vi "五参数水样测试.vi"(11 "启动参数":T1={"测量模式"="", "数据类型"="N"}) -> ()   [LabVIEW 2016, in "斯坦道原位多参数.lvlib"]
panel:
  out "Elapsed Time (s)":dbl caption="已用时间(s)"
  out "状态":string
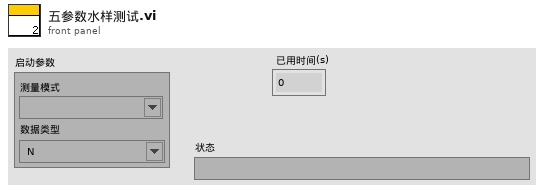
[diagram p1: front panel]
types:
  T1 = typedef "斯坦道原位多参数.lvlib/水样测试启动自定义输入参数.ctl" = cluster{"测量模式":string, "数据类型":string}
  T2 = cluster{"时间标识":timestamp, "设备":string, "日志信息":string, "流程参数":string}
  T3 = cluster{"水温":bool, "pH":bool, "DO":bool, "DOper":bool, "电导率":bool, "ORP":bool, "浊度":bool, "叶绿素a":bool, "藻密度":bool}
  T4 = typedef "原位多参数全参数字段定义.ctl" = cluster{"时间":timestamp, "水温":dbl, "pH":dbl, "DO":dbl, "DO%":dbl, "电导率":dbl, "ORP":dbl, "浊度":dbl, "叶绿素a":dbl, "藻密度":dbl}
  T5 = cluster{"系统时间":timestamp, "工作状态":u16, "测量模式":u16, "告警代码":enum16{"无告警", "缺试剂告警", "缺水样告警", "缺蒸馏水告警", "缺标液告警", "仪表漏液告警", "标定异常告警", "超量程告警", "加热异常", "低试剂预警", "超上限告警", "超下限告警", "仪表内部其他异常", "滴定异常告警", "电极异常告警", "量程切换告警", "参数设置告警", "PH电极电位异常", "电导率电极异常", "浊度光度异常", "溶解氧电极异常", "溶解氧光强异常", "温度异常告警", "PH异常告警", "溶解氧异常告警", "电导率异常告警", "浊度异常告警", "叶绿素异常告警", "藻密度异常告警", "蓝绿藻异常告警", "ORP异常告警", "氨氮异常告警", "清洁刷异常告警", "SD卡异常告警", "蓝牙异常告警", "Wifi异常告警", "流程异常告警"}, "故障代码":enum16{"无故障", "电机故障", "温度故障", "通讯故障", "滴定故障"}, "日志代码":u16, "软件版本":string}
  T6 = cluster{"水温":dbl, "pH":dbl, "DO":dbl, "Cond":dbl, "Turb":dbl, "叶绿素":dbl, "藻密度":dbl, "蓝绿藻":dbl, "ORP":dbl, "NH3N":dbl}
  T7 = cluster{"因子编码":string, "单位":string, "标样参考值":sgl, "水样数据时间":timestamp, "水样实测值":sgl, "水样数据标识":string, "K":sgl, "B":sgl, "T":sgl, "H":sgl, "水深":sgl, "探头温度":sgl, "信号值":sgl}
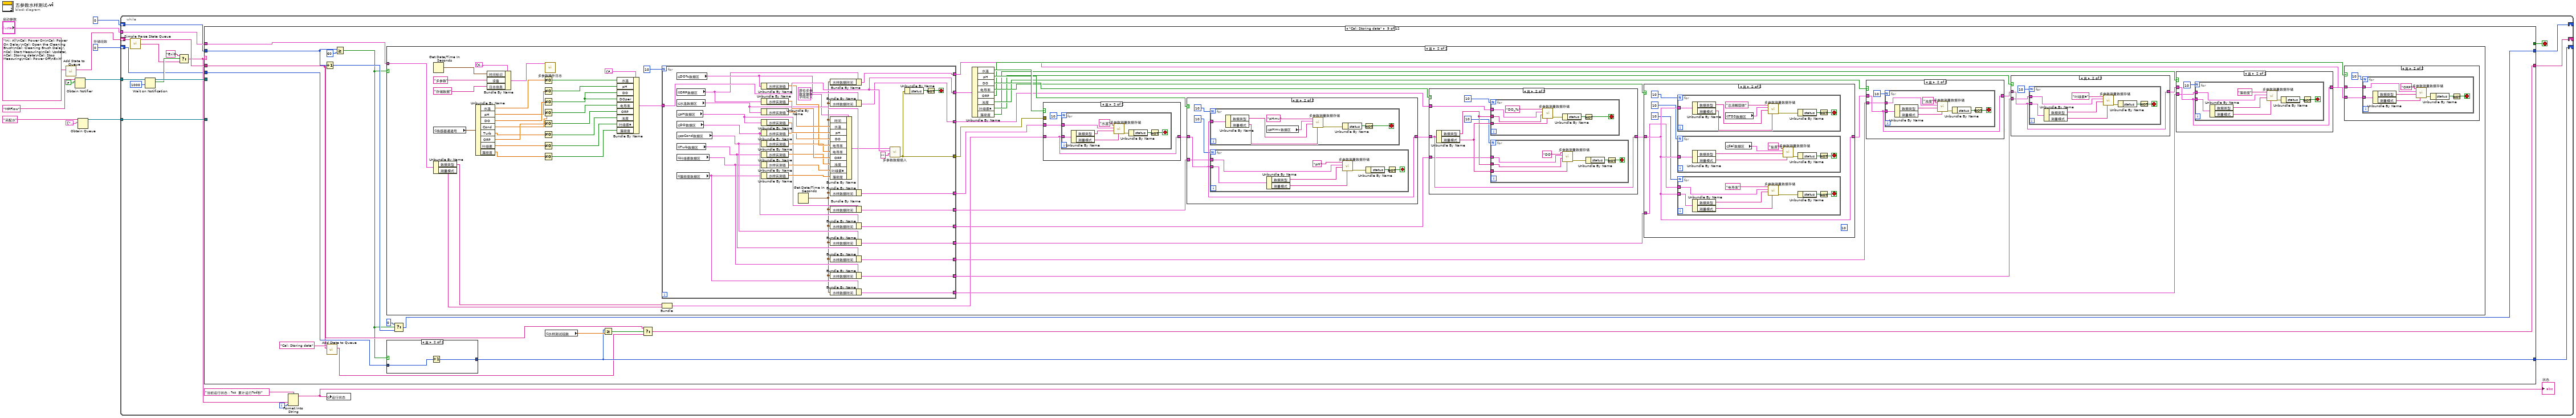
[diagram p0: block diagram]
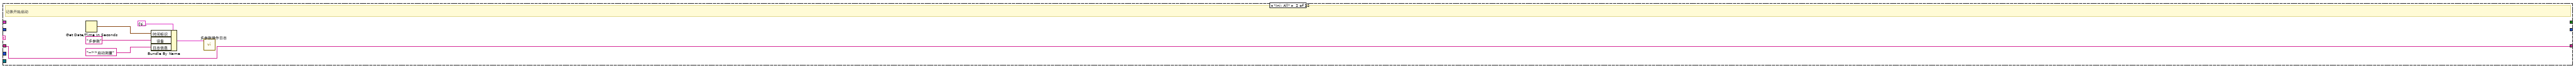
[diagram p3: hidden frame]
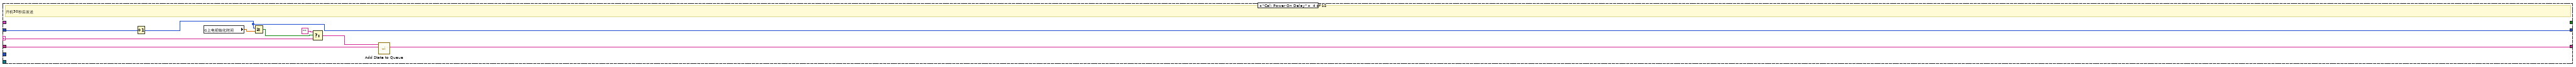
[diagram p5: hidden frame]
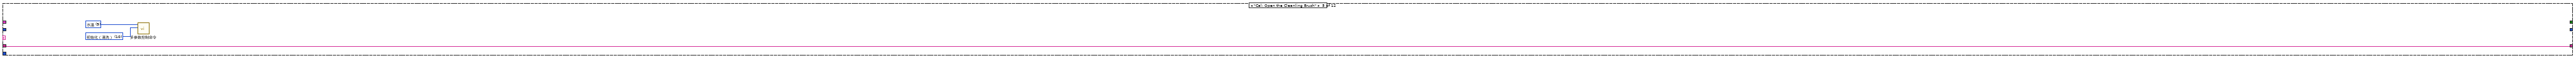
[diagram p6: hidden frame]
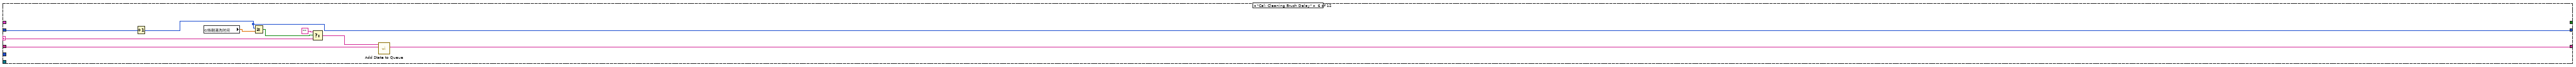
[diagram p7: hidden frame]
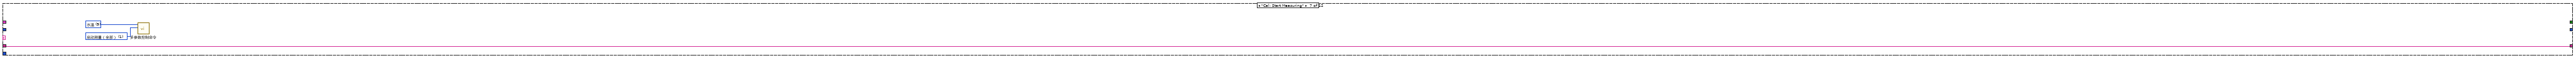
[diagram p8: hidden frame]
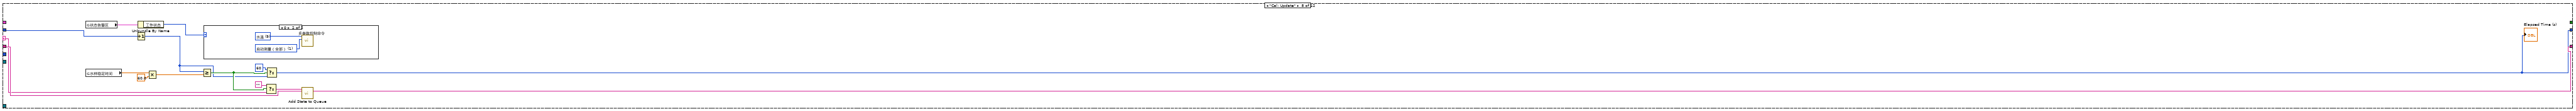
[diagram p9: hidden frame]
diagram:
  w1 = 0  # 存储组数
  n1 = call "Add State to Queue.vi"("State(s) In (\"\")"="Ini: All\nCal: Power On\nCal: Power On Delay\nCal: Open the Cleaning Brush\nCal: Cleaning Brush Delay\nCal: Start Measuring\nCal: Update\nCal: Storing data\nCal: Stop Measuring\nCal: Power Off\nExit" ("State(s) In (\"\")")) -> ("States Out"=w10:string)  [unwired: 14 in]
  n2 = Obtain Notifier(name (unnamed)="MPFlow" ("名称（未命名）"), notification data type=FALSE) -> (notifier out=w4:refnum<notifier>)  [unwired: 2 in, 2 out]
  n3 = Obtain Queue(name (unnamed)="采配水" ("名称（未命名）"), element data type=cluster{"命令":string, "数据":variant} {"命令"="", "数据"=variant}) -> (queue out=w5:refnum<queue>)  [unwired: 3 in, 2 out]
  n4 = while {
    shift-right: [w29] -> _
    shift-left: w10 -> [w31]
    tunnel: w5 -> [w28]
    tunnel: w4 -> [w27]
    tunnel: "启动参数" -> [w26]
    shift-right: [w14] -> _
    shift-left: 0 -> [w15]
    shift-right: [w13] -> _
    shift-left: w1 -> [w12]
    i -> [w24]
    stop <- w22 stop-if-true
    n5 = call "Simple Parse State Queue.vi"("State Queue"=w31) -> ("Remain States"=w30:string, "Next State"=w17:string)  [unwired: 13 in]
    n6 = Wait on Notification(notifier=w27, timeout in ms (-1)=1000 ("超时毫秒(-1)")) -> (notifier out=w21:refnum<notifier>, notification=w19:bool)  [unwired: 2 in, 2 out]
    n7 = Select(t="Exit" ("State(s) In (\"\")"), s=w19, f=w17) -> (s? t:f=w16:string)
    n8 = case shown="\"Cal: Storing data\"" w16 {
      selector: w16 -> [_ _ _ w46 _ w56 _ w74 _ _ _ _]
      tunnel: w30 -> [w32 w38 w39 w48 w51 w60 w61 w75 w87 w321 w330 w333]
      tunnel: [w32 w38 w39 w47 w51 w59 w61 w71 w89 w321 w330 w333] -> w29
      tunnel: w28 -> [_ _ _ _ _ _ _ _ _ _ _ w332]
      tunnel: w21 -> [_ _ _ _ _ _ _ _ _ _ _ w331]
      tunnel: w26 -> [_ _ _ _ _ _ _ _ w95 _ _ _]
      tunnel: [_ _ _ _ _ _ _ _ _ _ _ TRUE] -> w22
      tunnel: w15 -> [_ _ _ w43 _ w55 _ w70 w86 _ _ _]
      tunnel: [_ _ _ w42 _ w54 _ w65 w83 _ _ _] -> w14
      tunnel: w12 -> [_ _ _ _ _ _ _ _ w94 _ _ _]
      tunnel: [_ _ _ _ _ _ _ _ w91 _ _ _] -> w13
      frame Default {
      }
      frame "Ini: All" {
        # "记录开始启动"
        n9 = Get Date/Time In Seconds() -> (seconds since 1Jan1904=w34:timestamp)
        n10 = Bundle By Name(cluster=T2 {"时间标识"=timestamp(0 s since 1904-01-01), "设备"="", "日志信息"="", "流程参数"=""} ("data in"), "时间标识"=w34, "设备"="多参数", "日志信息"="-->>启动测量") -> (w35:T2)
        n11 = call "多参数操作日志.vi"("data"=w35) -> ()  [unwired: 10 in, 1 out]
      }
      frame "Cal: Power On" {
      }
      frame "Cal: Power On Delay" {
        # "开机30秒后发送"
        n12 = Increment(x=w43) -> (x+1=w42:i32)
        n13 = global read "多参数断电保存全局变量.vi" "上电初始化时间"() -> (w40:dbl)
        n14 = Greater Or Equal?(x=w42, y=w40) -> (x >= y?=w41:bool)
        n15 = Select(t="", s=w41, f=w46) -> (s? t:f=w44:string)
        n16 = call "Add State to Queue.vi"("State(s) In Front (\"\")"=w44, "State(s) In (\"\")"=w48) -> ("States Out"=w47:string)  [unwired: 13 in]
      }
      frame "Cal: Open the Cleanling Brush" {
        w50 = u16 10 items=["启动测量（全部）"=1, "初始化（清洗）"=10, "停止测量（全部）"=11, "校时"=13, "启动测量（单个传感器）"=19, "停止测量（单个传感器）"=20] ("控制命令")
        w49 = u16 9 items=["氨氮"=3, "水温"=9, "pH值"=10, "溶解氧"=11, "电导率"=12, "浊度"=13, "叶绿素a"=14, "藻密度"=15, "蓝绿藻"=16, "氧化还原电位"=17, "溶解氧%"=18, "盐度"=19] ("站号")
        n17 = call "多参数控制命令.vi"("控制命令"=w50, "站号"=w49) -> ()  [unwired: 9 in, 1 out]
      }
      frame "Cal: Cleaning Brush Delay" {
        n18 = Increment(x=w55) -> (x+1=w54:i32)
        n19 = global read "多参数断电保存全局变量.vi" "转刷清洗时间"() -> (w52:dbl)
        n20 = Greater Or Equal?(x=w54, y=w52) -> (x >= y?=w53:bool)
        n21 = Select(t="", s=w53, f=w56) -> (s? t:f=w57:string)
        n22 = call "Add State to Queue.vi"("State(s) In Front (\"\")"=w57, "State(s) In (\"\")"=w60) -> ("States Out"=w59:string)  [unwired: 13 in]
      }
      frame "Cal: Start Measuring" {
        w63 = u16 1 items=["启动测量（全部）"=1, "初始化（清洗）"=10, "停止测量（全部）"=11, "校时"=13, "启动测量（单个传感器）"=19, "停止测量（单个传感器）"=20] ("控制命令")
        w62 = u16 9 items=["氨氮"=3, "水温"=9, "pH值"=10, "溶解氧"=11, "电导率"=12, "浊度"=13, "叶绿素a"=14, "藻密度"=15, "蓝绿藻"=16, "氧化还原电位"=17, "溶解氧%"=18, "盐度"=19] ("站号")
        n23 = call "多参数控制命令.vi"("控制命令"=w63, "站号"=w62) -> ()  [unwired: 9 in, 1 out]
      }
      frame "Cal: Update" {
        n24 = global read "多参数全局变量.vi" "状态告警区"() -> (w77:T5)
        n25 = global read "多参数断电保存全局变量.vi" "水样稳定时间"() -> (w68:dbl)
        n26 = Increment(x=w70) -> (x+1=w66:i32)
        n27 = Unbundle By Name(w77) -> ("工作状态"=w78:u16)
        n28 = Multiply(x=w68, y=60.0) -> (x*y=w69:dbl)
        n29 = Greater Or Equal?(x=w66, y=w69) -> (x >= y?=w67:bool)
        n30 = case shown="0" w78 {
          frame Default {
          }
          frame 0 {
            w79 = u16 1 items=["启动测量（全部）"=1, "初始化（清洗）"=10, "停止测量（全部）"=11, "校时"=13, "启动测量（单个传感器）"=19, "停止测量（单个传感器）"=20] ("控制命令")
            w80 = u16 9 items=["氨氮"=3, "水温"=9, "pH值"=10, "溶解氧"=11, "电导率"=12, "浊度"=13, "叶绿素a"=14, "藻密度"=15, "蓝绿藻"=16, "氧化还原电位"=17, "溶解氧%"=18, "盐度"=19] ("站号")
            n31 = call "多参数控制命令.vi"("控制命令"=w79, "站号"=w80) -> ()  [unwired: 9 in, 1 out]
          }
        }
        n32 = Select(t="", s=w67, f=w74) -> (s? t:f=w73:string)
        n33 = Select(t=60, s=w67, f=w66) -> (s? t:f=w65:i32)
        "Elapsed Time (s)" <- w65
        n34 = call "Add State to Queue.vi"("State(s) In Front (\"\")"=w73, "State(s) In (\"\")"=w75) -> ("States Out"=w71:string)  [unwired: 13 in]
      }
      frame "Cal: Storing data" {
        n35 = Increment(x=w86) -> (x+1=w84:i32)
        n36 = call "Add State to Queue.vi"("State(s) In Front (\"\")"="Cal: Storing data" ("State(s) In Front (\"\")"), "State(s) In (\"\")"=w87) -> ("States Out"=w88:string)  [unwired: 13 in]
        n37 = Greater Or Equal?(x=w86, y=60) -> (x >= y?=w81:bool)
        n38 = case shown="真" w81 {
          tunnel: w95 -> [_ w139]
          frame False {
          }
          frame True {
            n39 = Get Date/Time In Seconds() -> (seconds since 1Jan1904=w148:timestamp)
            n40 = global read "多参数全局变量.vi" "传感器通道号"() -> (w121:T6)
            n41 = Unbundle By Name(w139) -> ("数据类型"=w140:string, "测量模式"=w141:string)
            n42 = Unbundle By Name(w121) -> ("水温"=w119:dbl, "pH"=w122:dbl, "DO"=w124:dbl, "Cond"=w126:dbl, "Turb"=w128:dbl, "ORP"=w130:dbl, "叶绿素"=w132:dbl, "藻密度"=w133:dbl)
            n43 = Bundle By Name(cluster=T2 {"时间标识"=timestamp(0 s since 1904-01-01), "设备"="", "日志信息"="", "流程参数"=""} ("data in"), "时间标识"=w148, "设备"="多参数", "日志信息"="存储数据") -> (w149:T2)
            n44 = Not Equal To 0?(x=w119) -> (x != 0?=w120:bool)
            n45 = Not Equal To 0?(x=w122) -> (x != 0?=w123:bool)
            n46 = Not Equal To 0?(x=w124) -> (x != 0?=w125:bool)
            n47 = Not Equal To 0?(x=w126) -> (x != 0?=w127:bool)
            n48 = Not Equal To 0?(x=w130) -> (x != 0?=w131:bool)
            n49 = Not Equal To 0?(x=w128) -> (x != 0?=w129:bool)
            n50 = Not Equal To 0?(x=w132) -> (x != 0?=w134:bool)
            n51 = Not Equal To 0?(x=w133) -> (x != 0?=w135:bool)
            n52 = call "多参数操作日志.vi"("data"=w149) -> ()  [unwired: 10 in, 1 out]
            n53 = Bundle By Name(cluster=T3 {"水温"=FALSE, "pH"=FALSE, "DO"=FALSE, "DOper"=FALSE, "电导率"=FALSE, "ORP"=FALSE, "浊度"=FALSE, "叶绿素a"=FALSE, "藻密度"=FALSE} ("columns enable"), "水温"=w120, "pH"=w123, "DO"=w125, "DOper"=w125, "电导率"=w127, "ORP"=w131, "浊度"=w129, "叶绿素a"=w134, "藻密度"=w135) -> (w117:T3)
            n54 = for {
              N: 10 -> [_]
              tunnel: [w186] -> w136
              tunnel: w117 -> [w185]
              tunnel: [w185] -> w108
              tunnel: [w161] -> w107
              tunnel: [w160] -> w106
              tunnel: [w159] -> w105
              tunnel: [w162] -> w104
              tunnel: [w158] -> w103
              tunnel: [w166] -> w102
              tunnel: [w163] -> w101
              tunnel: [w164] -> w100
              tunnel: [w165] -> w99
              stop <- w187 stop-if-true
              n55 = global read "多参数全局变量.vi" "DO%数据区"() -> (w172:T7)
              n56 = global read "多参数全局变量.vi" "ORP数据区"() -> (w170:T7)
              n57 = global read "多参数全局变量.vi" "水温数据区"() -> (w175:T7)
              n58 = global read "多参数全局变量.vi" "pH数据区"() -> (w174:T7)
              n59 = global read "多参数全局变量.vi" "DO数据区"() -> (w173:T7)
              n60 = global read "多参数全局变量.vi" "spCond数据区"() -> (w171:T7)
              n61 = global read "多参数全局变量.vi" "Turb数据区"() -> (w169:T7)
              n62 = global read "多参数全局变量.vi" "叶绿素数据区"() -> (w168:T7)
              n63 = global read "多参数全局变量.vi" "藻密度数据区"() -> (w167:T7)
              n64 = Unbundle By Name(w172) -> ("水样实测值"=w181:sgl)
              n65 = Unbundle By Name(w170) -> ("水样实测值"=w179:sgl)
              n66 = Unbundle By Name(w175) -> ("水样实测值"=w184:sgl)
              n67 = Unbundle By Name(w174) -> ("水样实测值"=w183:sgl)
              n68 = Unbundle By Name(w173) -> ("水样实测值"=w182:sgl)
              n69 = Unbundle By Name(w171) -> ("水样实测值"=w180:sgl)
              n70 = Unbundle By Name(w169) -> ("水样实测值"=w178:sgl)
              n71 = Unbundle By Name(w168) -> ("水样实测值"=w177:sgl)
              n72 = Unbundle By Name(w167) -> ("水样实测值"=w176:sgl)
              n73 = Get Date/Time In Seconds() -> (seconds since 1Jan1904=w157:timestamp)
              n74 = Bundle By Name(cluster=w170, "水样数据时间"=w157) -> (w166:T7)
              n75 = Bundle By Name(cluster=w172, "水样数据时间"=w157) -> (w162:T7)
              n76 = Bundle By Name(cluster=T4 {"时间"=timestamp(0 s since 1904-01-01), "水温"=0.0, "pH"=0.0, "DO"=0.0, "DO%"=0.0, "电导率"=0.0, "ORP"=0.0, "浊度"=0.0, "叶绿素a"=0.0, "藻密度"=0.0} ("data in"), "时间"=w157, "水温"=w184, "pH"=w183, "DO"=w182, "电导率"=w181, "电导率"=w180, "ORP"=w179, "浊度"=w178, "叶绿素a"=w177, "藻密度"=w176) -> (w155:T4)
              n77 = Bundle By Name(cluster=w175, "水样数据时间"=w157) -> (w161:T7)
              n78 = Bundle By Name(cluster=w174, "水样数据时间"=w157) -> (w160:T7)
              n79 = Bundle By Name(cluster=w173, "水样数据时间"=w157) -> (w159:T7)
              n80 = Bundle By Name(cluster=w171, "水样数据时间"=w157) -> (w158:T7)
              n81 = Bundle By Name(cluster=w169, "水样数据时间"=w157) -> (w163:T7)
              n82 = Bundle By Name(cluster=w168, "水样数据时间"=w157) -> (w164:T7)
              n83 = Bundle By Name(cluster=w167, "水样数据时间"=w157) -> (w165:T7)
              n84 = call "多参数数据插入.vi"("编号"="", "columns enable"=w185, "data in"=w155) -> ("error out"=w186:errorcluster)  [unwired: 8 in]
              n85 = Unbundle By Name(w186) -> ("status"=w188:bool)
              n86 = Not(x=w188) -> (.not. x?=w187:bool)
            }
            n87 = Bundle("数据类型"=w140, "测量模式"=w141) -> (w142:cluster{"数据类型":string, "测量模式":string})  [unwired: 1 in]
            n88 = Unbundle By Name(w108) -> ("水温"=w116:bool, "pH"=w115:bool, "DO"=w114:bool, "电导率"=w113:bool, "ORP"=w109:bool, "浊度"=w112:bool, "叶绿素a"=w111:bool, "藻密度"=w110:bool)
            n89 = case shown="真" w116 {
              tunnel: w142 -> [w309 w312]
              tunnel: [w309 w312] -> w143
              tunnel: w136 -> [_ _]
              tunnel: w107 -> [_ w310]
              frame False {
              }
              frame True {
                n90 = for {
                  N: 10 -> [_]
                  tunnel: w312 -> [w320]
                  tunnel: w310 -> [w315]
                  stop <- w317 stop-if-true
                  n91 = Unbundle By Name(w320) -> ("数据类型"=w314:string, "测量模式"=w313:string)
                  n92 = call "多参数测量数据存储.vi"("测量模式"=w313, "数据类型"=w314, "数据区"=w315, "table输入"="水温") -> ("error out"=w319:errorcluster)  [unwired: 7 in]
                  n93 = Unbundle By Name(w319) -> ("status"=w318:bool)
                  n94 = Not(x=w318) -> (.not. x?=w317:bool)
                }
              }
            }
            n95 = case shown="真" w115 {
              tunnel: w143 -> [w288 w292]
              tunnel: [w288 w292] -> w145
              tunnel: w106 -> [_ w289]
              frame False {
              }
              frame True {
                n96 = for {
                  N: 10 -> [_]
                  tunnel: w292 -> [w300]
                  stop <- w297 stop-if-true
                  n97 = Unbundle By Name(w300) -> ("数据类型"=w294:string, "测量模式"=w293:string)
                  n98 = global read "多参数全局变量.vi" "pHmv数据区"() -> (w295:T7)
                  n99 = call "多参数测量数据存储.vi"("测量模式"=w293, "数据类型"=w294, "数据区"=w295, "table输入"="pHmv") -> ("error out"=w299:errorcluster)  [unwired: 7 in]
                  n100 = Unbundle By Name(w299) -> ("status"=w298:bool)
                  n101 = Not(x=w298) -> (.not. x?=w297:bool)
                }
                n102 = for {
                  N: 10 -> [_]
                  tunnel: w292 -> [w308]
                  tunnel: w289 -> [w301]
                  stop <- w305 stop-if-true
                  n103 = Unbundle By Name(w308) -> ("数据类型"=w303:string, "测量模式"=w302:string)
                  n104 = call "多参数测量数据存储.vi"("测量模式"=w302, "数据类型"=w303, "数据区"=w301, "table输入"="pH") -> ("error out"=w307:errorcluster)  [unwired: 7 in]
                  n105 = Unbundle By Name(w307) -> ("status"=w306:bool)
                  n106 = Not(x=w306) -> (.not. x?=w305:bool)
                }
              }
            }
            n107 = case shown="真" w114 {
              tunnel: [w266 w273] -> w144
              tunnel: w145 -> [w266 w273]
              tunnel: w105 -> [_ w268]
              tunnel: w104 -> [_ w267]
              frame False {
              }
              frame True {
                n108 = Unbundle By Name(w273) -> ("数据类型"=w271:string, "测量模式"=w272:string)
                n109 = for {
                  N: 10 -> [_]
                  tunnel: w272 -> [w281]
                  tunnel: w271 -> [w282]
                  tunnel: w267 -> [w283]
                  stop <- w285 stop-if-true
                  n110 = call "多参数测量数据存储.vi"("测量模式"=w281, "数据类型"=w282, "数据区"=w283, "table输入"="DO_%") -> ("error out"=w287:errorcluster)  [unwired: 7 in]
                  n111 = Unbundle By Name(w287) -> ("status"=w286:bool)
                  n112 = Not(x=w286) -> (.not. x?=w285:bool)
                }
                n113 = for {
                  N: 10 -> [_]
                  tunnel: w272 -> [w275]
                  tunnel: w271 -> [w276]
                  tunnel: w268 -> [w274]
                  stop <- w278 stop-if-true
                  n114 = call "多参数测量数据存储.vi"("测量模式"=w275, "数据类型"=w276, "数据区"=w274, "table输入"="DO") -> ("error out"=w280:errorcluster)  [unwired: 7 in]
                  n115 = Unbundle By Name(w280) -> ("status"=w279:bool)
                  n116 = Not(x=w279) -> (.not. x?=w278:bool)
                }
              }
            }
            n117 = case shown="真" w113 {
              tunnel: w144 -> [w236 w241]
              tunnel: [w236 w241] -> w146
              tunnel: w103 -> [_ w237]
              frame False {
              }
              frame True {
                (unwired) 10
                n118 = for {
                  N: 10 -> [_]
                  tunnel: w241 -> [w249]
                  stop <- w246 stop-if-true
                  n119 = Unbundle By Name(w249) -> ("数据类型"=w243:string, "测量模式"=w242:string)
                  n120 = global read "多参数全局变量.vi" "TDS数据区"() -> (w244:T7)
                  n121 = call "多参数测量数据存储.vi"("测量模式"=w242, "数据类型"=w243, "数据区"=w244, "table输入"="总溶解固体") -> ("error out"=w248:errorcluster)  [unwired: 7 in]
                  n122 = Unbundle By Name(w248) -> ("status"=w247:bool)
                  n123 = Not(x=w247) -> (.not. x?=w246:bool)
                }
                n124 = for {
                  N: 10 -> [_]
                  tunnel: w241 -> [w265]
                  stop <- w262 stop-if-true
                  n125 = Unbundle By Name(w265) -> ("数据类型"=w259:string, "测量模式"=w258:string)
                  n126 = global read "多参数全局变量.vi" "Sal数据区"() -> (w260:T7)
                  n127 = call "多参数测量数据存储.vi"("测量模式"=w258, "数据类型"=w259, "数据区"=w260, "table输入"="盐度") -> ("error out"=w264:errorcluster)  [unwired: 7 in]
                  n128 = Unbundle By Name(w264) -> ("status"=w263:bool)
                  n129 = Not(x=w263) -> (.not. x?=w262:bool)
                }
                n130 = for {
                  N: 10 -> [_]
                  tunnel: w241 -> [w257]
                  tunnel: w237 -> [w252]
                  stop <- w254 stop-if-true
                  n131 = Unbundle By Name(w257) -> ("数据类型"=w251:string, "测量模式"=w250:string)
                  n132 = call "多参数测量数据存储.vi"("测量模式"=w250, "数据类型"=w251, "数据区"=w252, "table输入"="电导率") -> ("error out"=w256:errorcluster)  [unwired: 7 in]
                  n133 = Unbundle By Name(w256) -> ("status"=w255:bool)
                  n134 = Not(x=w255) -> (.not. x?=w254:bool)
                }
              }
            }
            n135 = case shown="真" w112 {
              tunnel: w146 -> [w224 w227]
              tunnel: [w224 w227] -> w152
              tunnel: w101 -> [_ w225]
              frame False {
              }
              frame True {
                n136 = for {
                  N: 10 -> [_]
                  tunnel: w227 -> [w235]
                  tunnel: w225 -> [w230]
                  stop <- w232 stop-if-true
                  n137 = Unbundle By Name(w235) -> ("数据类型"=w229:string, "测量模式"=w228:string)
                  n138 = call "多参数测量数据存储.vi"("测量模式"=w228, "数据类型"=w229, "数据区"=w230, "table输入"="浊度") -> ("error out"=w234:errorcluster)  [unwired: 7 in]
                  n139 = Unbundle By Name(w234) -> ("status"=w233:bool)
                  n140 = Not(x=w233) -> (.not. x?=w232:bool)
                }
              }
            }
            n141 = case shown="真" w111 {
              tunnel: w152 -> [w212 w215]
              tunnel: [w212 w215] -> w153
              tunnel: w100 -> [_ w213]
              frame False {
              }
              frame True {
                n142 = for {
                  N: 10 -> [_]
                  tunnel: w215 -> [w223]
                  tunnel: w213 -> [w216]
                  stop <- w220 stop-if-true
                  n143 = Unbundle By Name(w223) -> ("数据类型"=w219:string, "测量模式"=w218:string)
                  n144 = call "多参数测量数据存储.vi"("测量模式"=w218, "数据类型"=w219, "数据区"=w216, "table输入"="叶绿素a") -> ("error out"=w222:errorcluster)  [unwired: 7 in]
                  n145 = Unbundle By Name(w222) -> ("status"=w221:bool)
                  n146 = Not(x=w221) -> (.not. x?=w220:bool)
                }
              }
            }
            n147 = case shown="真" w110 {
              tunnel: w153 -> [w200 w203]
              tunnel: [w200 w203] -> w138
              tunnel: w99 -> [_ w201]
              frame False {
              }
              frame True {
                n148 = for {
                  N: 10 -> [_]
                  tunnel: w203 -> [w211]
                  tunnel: w201 -> [w204]
                  stop <- w208 stop-if-true
                  n149 = Unbundle By Name(w211) -> ("数据类型"=w206:string, "测量模式"=w205:string)
                  n150 = call "多参数测量数据存储.vi"("测量模式"=w205, "数据类型"=w206, "数据区"=w204, "table输入"="藻密度") -> ("error out"=w210:errorcluster)  [unwired: 7 in]
                  n151 = Unbundle By Name(w210) -> ("status"=w209:bool)
                  n152 = Not(x=w209) -> (.not. x?=w208:bool)
                }
              }
            }
            n153 = case shown="真" w109 {
              tunnel: w138 -> [_ w191]
              tunnel: w102 -> [_ w189]
              frame False {
              }
              frame True {
                n154 = for {
                  N: 10 -> [_]
                  tunnel: w191 -> [w199]
                  tunnel: w189 -> [w194]
                  stop <- w196 stop-if-true
                  n155 = Unbundle By Name(w199) -> ("数据类型"=w193:string, "测量模式"=w192:string)
                  n156 = call "多参数测量数据存储.vi"("测量模式"=w192, "数据类型"=w193, "数据区"=w194, "table输入"="ORP") -> ("error out"=w198:errorcluster)  [unwired: 7 in]
                  n157 = Unbundle By Name(w198) -> ("status"=w197:bool)
                  n158 = Not(x=w197) -> (.not. x?=w196:bool)
                }
              }
            }
          }
        }
        n159 = case shown="真" w81 {
          tunnel: w94 -> [w96 w98]
          tunnel: [w96 w97] -> w91
          frame False {
          }
          frame True {
            n160 = Increment(x=w98) -> (x+1=w97:i32)
          }
        }
        n161 = Select(t=0, s=w81, f=w84) -> (s? t:f=w83:i32)
        n162 = global read "多参数断电保存全局变量.vi" "水样测试组数"() -> (w92:dbl)
        n163 = Greater Or Equal?(x=w91, y=w92) -> (x >= y?=w90:bool)
        n164 = Select(t=w87, s=w90, f=w88) -> (s? t:f=w89:string)
      }
      frame "Cal: Stop Measuring" {
        n165 = Get Date/Time In Seconds() -> (seconds since 1Jan1904=w324:timestamp)
        n166 = flat-sequence {
          frame #0 {
            w327 = u16 11 items=["启动测量（全部）"=1, "初始化（清洗）"=10, "停止测量（全部）"=11, "校时"=13, "启动测量（单个传感器）"=19, "停止测量（单个传感器）"=20] ("控制命令")
            w328 = u16 9 items=["氨氮"=3, "水温"=9, "pH值"=10, "溶解氧"=11, "电导率"=12, "浊度"=13, "叶绿素a"=14, "藻密度"=15, "蓝绿藻"=16, "氧化还原电位"=17, "溶解氧%"=18, "盐度"=19] ("站号")
            n167 = call "多参数控制命令.vi"("控制命令"=w327, "站号"=w328) -> ()  [unwired: 9 in, 1 out]
          }
          frame #1 {
            n168 = Wait (ms)(milliseconds to wait=u32 2000 ("等待时间（毫秒）")) -> ()  [unwired: 1 out]
          }
        }
        n169 = Bundle By Name(cluster=T2 {"时间标识"=timestamp(0 s since 1904-01-01), "设备"="", "日志信息"="", "流程参数"=""} ("data in"), "时间标识"=w324, "设备"="多参数", "日志信息"="-->>停止测量") -> (w323:T2)
        n170 = call "多参数操作日志.vi"("data"=w323) -> ()  [unwired: 10 in, 1 out]
      }
      frame "Cal: Power Off" {
      }
      frame "Exit" {
        n171 = Release Notifier(notifier=w331) -> ()  [unwired: 2 in, 3 out]
        n172 = Release Queue(queue=w332) -> ()  [unwired: 2 in, 3 out]
      }
    }
    n173 = Format Into String(format string="当前运行状态：%s  累计运行%d秒" ("格式字符串"), w16, w24) -> (resulting string=w23:string)  [unwired: 2 in, 1 out]
    "状态" <- w23
    n174 = global write "多参数全局变量.vi" "运行状态"(w23) -> ()
  }
